vi "HW_Gantner_Get Valid Device IP.vi"() -> (2 "ip out":string caption="值")   [LabVIEW 2016]
uses:
  <vilib>/Utility/config.llb/Read Key (String).vi
  <vilib>/Utility/config.llb/NI_LVConfig.lvlib
panel:
  out "error out":errorcluster caption="错误输出"
  in  "error in":errorcluster caption="错误输入（无错误）"
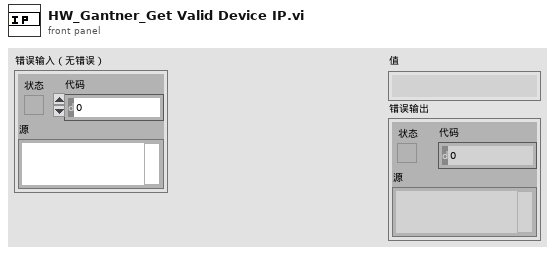
[diagram p1: front panel]
types:
  T1 = cluster{"DfltDataFolder":path, "ParaFolder":path, "SysCfg":path, "CHdef":path, "ModCfg":path, "DT Folder":path, "ErrorLog":path, "HBMlic":path, "HBMDriver":path}
  T2 = typedef "NI_LVConfig.lvlib/Config Data RefNum.ctl" = refnum<k1>
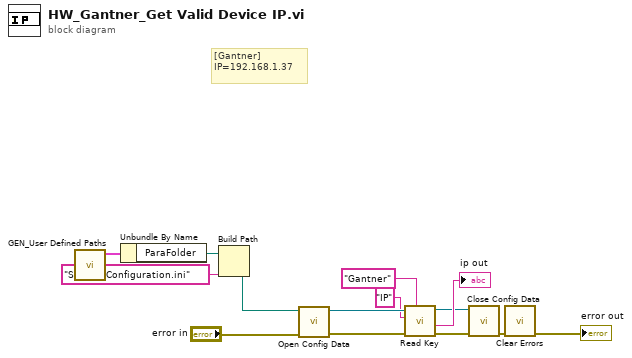
[diagram p0: block diagram]
diagram:
  # "[Gantner]\nIP=192.168.1.37"
  n1 = call "GEN_User Defined Paths.vi"() -> ("UserDefinedPath"=w9:T1)  [unwired: 11 in]
  n2 = Unbundle By Name(w9) -> ("ParaFolder"=w8:path)
  n3 = Build Path(base path=w8, name or relative path="System Configuration.ini" ("名称或相对路径")) -> (appended path=w6:path)
  n4 = call <vilib>:"Open Config Data.vi"("error in (no error)"="error in", "configuration file path"=w6) -> ("error out"=w13:errorcluster, "refnum"=w14:T2)  [unwired: 7 in, 1 out]
  n5 = call-poly <vilib>:"Read Key.vi"("section"="Gantner", "error in (no error)"=w13, "key"="IP" ("section"), "refnum"=w14) -> ("error out"=w4:errorcluster, "value"=→"ip out":string, "refnum out"=w5:T2)  [unwired: 4 in, 1 out]
  n6 = call <vilib>:"Close Config Data.vi"("error in (no error)"=w4, "refnum"=w5) -> ("error out"=w2:errorcluster)  [unwired: 8 in, 1 out]
  n7 = call <vilib>:"Clear Errors.vi"("error in (no error)"=w2) -> ("error out"=→"error out":errorcluster)  [unwired: 5 in, 1 out]
